vi "Create Mappings.vi"(8 "error in (no error)":errorcluster, 10 "data allocations":T2, 11 "Multiplexer configuration":refnum<class "Multiplexer configuration.lvclass">) -> (0 "error out":errorcluster, 3 "Mappings":T1[](array[typedef]))   [LabVIEW 2021, in "Multiplexer runtime.lvclass"]
uses:
  Multiplexer runtime.lvclass
  <vilib>/NI/Tag Bus Module Framework/channel/data tables.ctl
  <vilib>/NI/Tag Bus/dictionary/data dictionary.lvclass
  <vilib>/NI/Tag Bus/dictionary table pair.ctl
  <vilib>/NI/Tag Bus/table/data table.ctl
  Line Mappings.ctl
  configuration/Multiplexer configuration.lvclass
  configuration/Multiplexer configuration.lvclass/Multiplexer configuration.ctl
  <vilib>/NI/Tag Bus/tag/tag descriptor.lvclass/tag descriptor.ctl
  configuration/Read Lines.vi
  <vilib>/NI/Tag Bus/tag/read tag name.vi
  <vilib>/NI/Tag Bus/tag/read data type.vi
  <vilib>/NI/Tag Bus Module Framework/channel/TBM channel.lvclass
  C:/Program Files (x86)/National Instruments/LabVIEW 2021/vi.lib/NI/Tag Bus/tag/tag descriptor.lvclass
  <vilib>/NI/Tag Bus/dictionary/locate tag.vi
  <vilib>/NI/Tag Bus/table/data table.lvlib
  <vilib>/NI/Tag Bus/tag bus.lvlib
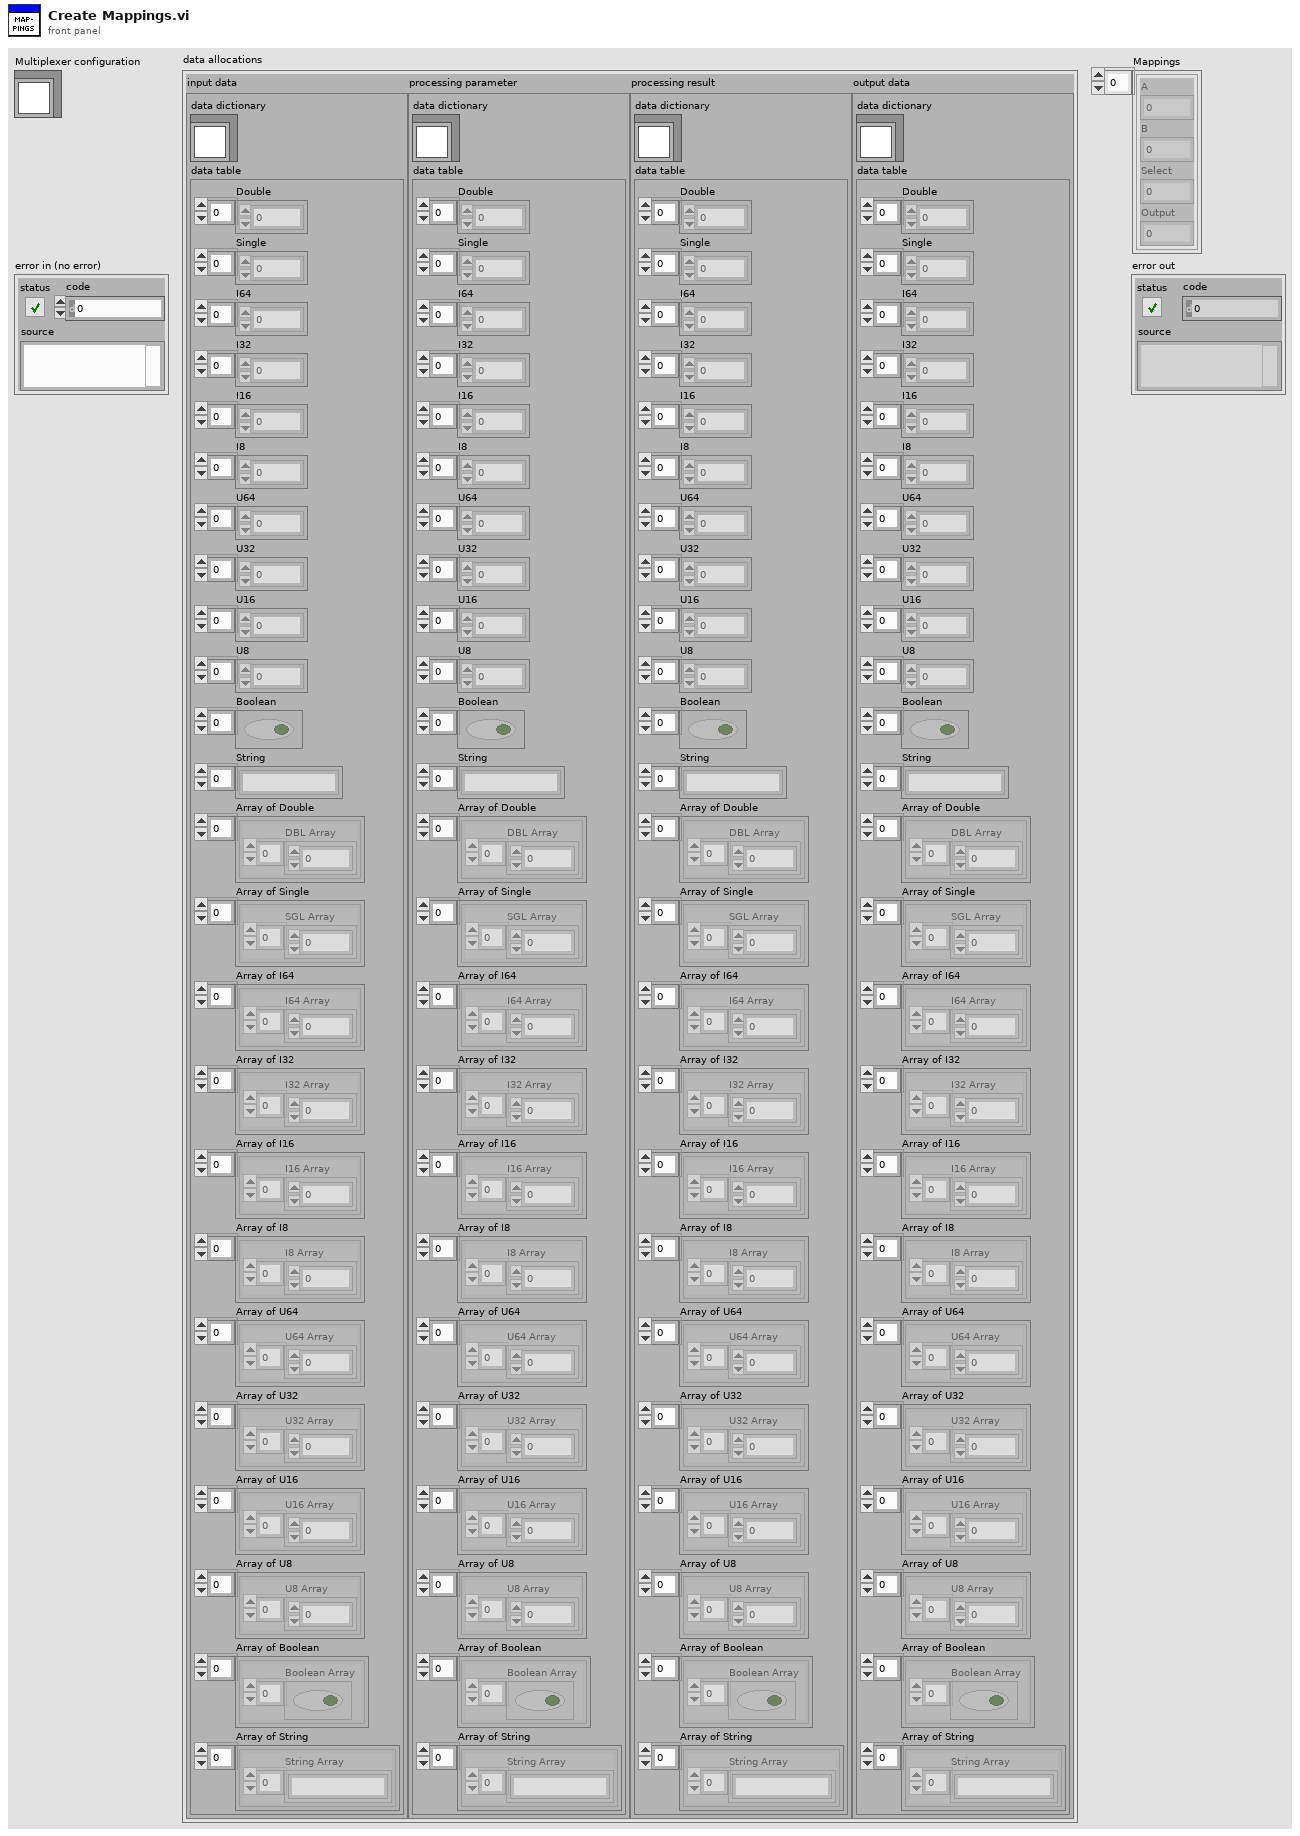
[diagram p1: front panel]
types:
  T1 = typedef "Multiplexer runtime.lvclass/Line Mappings.ctl" = cluster{"A":i32, "B":i32, "Select":i32, "Output":i32}
  T2 = typedef "TBM channel.lvclass/data tables.ctl" = cluster{"input data":T3, "processing parameter":T3, "processing result":T3, "output data":T3}
  T3 = typedef "tag bus.lvlib/dictionary table pair.ctl" = cluster{"data dictionary":refnum<class "data dictionary.lvclass">, "data table":T4}
  T4 = typedef "tag bus.lvlib/data table.lvlib/data table.ctl" = cluster{"Double":dbl[], "Single":sgl[], "I64":i64[], "I32":i32[], "I16":i16[], "I8":i8[], "U64":u64[], "U32":u32[], "U16":u16[], "U8":u8[], "Boolean":bool[], "String":string[], "Array of Double":cluster{"DBL Array":dbl[]}[], "Array of Single":cluster{"SGL Array":sgl[]}[], "Array of I64":cluster{"I64 Array":i64[]}[], "Array of I32":cluster{"I32 Array":i32[]}[], "Array of I16":cluster{"I16 Array":i16[]}[], "Array of I8":cluster{"I8 Array":i8[]}[], "Array of U64":cluster{"U64 Array":u64[]}[], "Array of U32":cluster{"U32 Array":u32[]}[], "Array of U16":cluster{"U16 Array":u16[]}[], "Array of U8":cluster{"U8 Array":u8[]}[], "Array of Boolean":cluster{"Boolean Array":bool[]}[], "Array of String":cluster{"String Array":string[]}[]}
  T5 = typedef "Multiplexer configuration.lvclass/Line.ctl" = cluster{"A":refnum<class "TBM channel.lvclass">, "B":refnum<class "TBM channel.lvclass">, "Select":refnum<class "TBM channel.lvclass">, "Output":refnum<class "TBM channel.lvclass">}
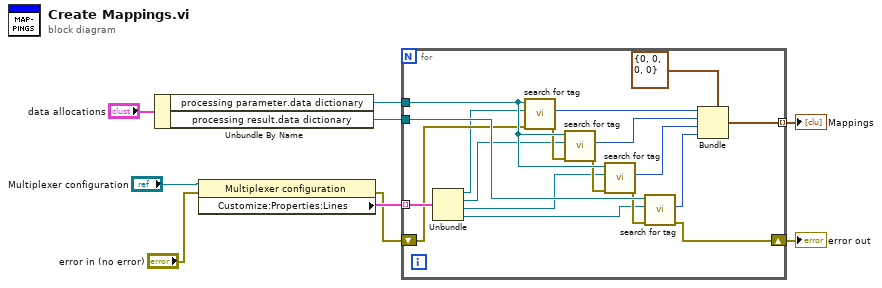
[diagram p0: block diagram]
diagram:
  n1 = Unbundle By Name("data allocations") -> ("processing parameter.data dictionary"=w4:refnum<class "data dictionary.lvclass">, "processing result.data dictionary"=w3:refnum<class "data dictionary.lvclass">)
  n2 = property class="Multiplexer configuration"(reference="Multiplexer configuration", error in="error in (no error)") -> (error out=w5:errorcluster, "Customize:Properties:Lines"=w7:T5[])  [unwired: 1 out]
  n3 = for {
    tunnel: w7 -> [w27] mode=indexing
    shift-right: [w21] -> w1
    shift-left: w5 -> [w20]
    tunnel: w4 -> [w25]
    tunnel: w3 -> [w26]
    tunnel: [w10] -> w2 mode=indexing
    n4 = Unbundle(w27) -> ("A"=w19:refnum<class "TBM channel.lvclass">, "B"=w18:refnum<class "TBM channel.lvclass">, "Select"=w17:refnum<class "TBM channel.lvclass">, "Output"=w16:refnum<class "TBM channel.lvclass">)
    n5 = call <vilib>:"search for tag.vi"("error in"=w20, "system tag"=w19, "data dictionary in"=w25) -> ("error out"=w24:errorcluster, "index"=w14:i32)  [unwired: 6 in, 1 out]
    n6 = call <vilib>:"search for tag.vi"("error in"=w24, "system tag"=w18, "data dictionary in"=w25) -> ("error out"=w23:errorcluster, "index"=w13:i32)  [unwired: 6 in, 1 out]
    n7 = call <vilib>:"search for tag.vi"("error in"=w23, "system tag"=w17, "data dictionary in"=w25) -> ("error out"=w22:errorcluster, "index"=w12:i32)  [unwired: 6 in, 1 out]
    n8 = call <vilib>:"search for tag.vi"("error in"=w22, "system tag"=w16, "data dictionary in"=w26) -> ("error out"=w21:errorcluster, "index"=w11:i32)  [unwired: 6 in, 1 out]
    n9 = Bundle(cluster=T1 {"A"=0, "B"=0, "Select"=0, "Output"=0} ("Line Mappings"), "A"=w14, "B"=w13, "Select"=w12, "Output"=w11) -> (w10:T1)
  }
  "Mappings" <- w2
  "error out" <- w1
